vi "FrameDownWithoutHEADLEN(SubVI).vi"(0 "input frame":string, 5 "frame length":u16) -> (2 "id":string, 3 "sn":string, 4 "op":string, 8 "ob":string, 10 "data":string, 13 "reverse":string, 14 "chksum":string, 15 "result":string)   [LabVIEW 2012]
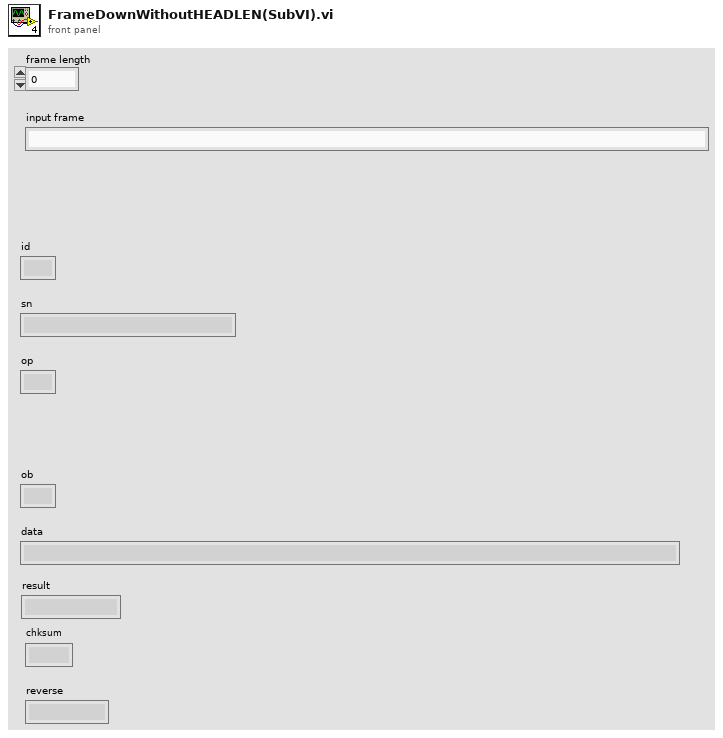
[diagram p1: front panel]
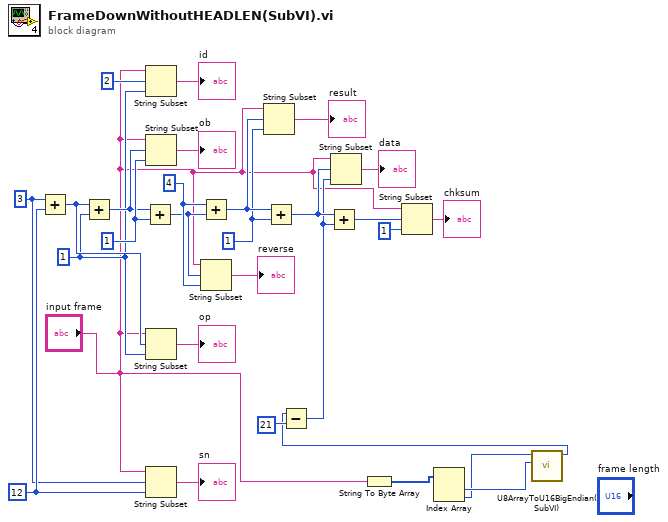
[diagram p0: block diagram]
diagram:
  w13 = 1
  w26 = 4
  w21 = 1
  w6 = 1
  w18 = 12
  w10 = 3
  n1 = Add(x=w10, y=w18) -> (x+y=w19:i32)
  n2 = Add(x=w19, y=w6) -> (x+y=w20:i32)
  n3 = Add(x=w20, y=w21) -> (x+y=w25:i32)
  n4 = String Subset(string="input frame", offset (0)=2, length (rest)=w6) -> (substring=→"id":string)
  n5 = String Subset(string="input frame", offset (0)=w20, length (rest)=w21) -> (substring=→"ob":string)
  n6 = String Subset(string="input frame", offset (0)=w19, length (rest)=w6) -> (substring=→"op":string)
  n7 = String Subset(string="input frame", offset (0)=w10, length (rest)=w18) -> (substring=→"sn":string)
  n8 = Add(x=w26, y=w25) -> (x+y=w14:i32)
  n9 = String Subset(string="input frame", offset (0)=w25, length (rest)=w26) -> (substring=→"reverse":string)
  n10 = String Subset(string="input frame", offset (0)=w14, length (rest)=w13) -> (substring=→"result":string)
  n11 = Add(x=w14, y=w13) -> (x+y=w12:i32)
  n12 = String To Byte Array(string="input frame") -> (unsigned byte array=w4:u8[])
  n13 = Index Array(array=w4) -> (element #1=w3:u8, element #2=w2:u8)  [unwired: 2 in]
  n14 = call "U8ArrayToU16BigEndian(SubVI).vi"("Numeric 7"=w3, "Numeric 6"=w2) -> ("Numeric 9"=w1:u16)  [unwired: 9 in]
  n15 = Subtract(x=w1, y=21) -> (x-y=w7:i32)
  n16 = Add(x=w12, y=w7) -> (x+y=w27:i32)
  n17 = String Subset(string="input frame", offset (0)=w12, length (rest)=w7) -> (substring=→"data":string)
  n18 = String Subset(string="input frame", offset (0)=w27, length (rest)=1) -> (substring=→"chksum":string)
